vi "write spi file type1.vi"(8 "milliseconds to wait":u32, 11 "addr/data":string[][](array[string])) -> (3 "res":bool)   [LabVIEW 2018]
uses:
  Dll1_x64_191014_0/Dll1_x64_191014_0.lvlib
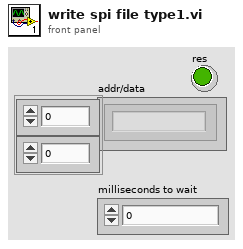
[diagram p1: front panel]
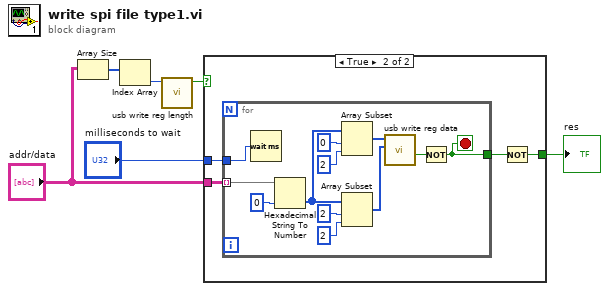
[diagram p0: block diagram]
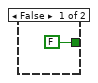
[diagram p2: hidden frame]
diagram:
  n1 = Array Size(array="addr/data") -> (size(s)=w5:i32[])
  n2 = Index Array(array=w5) -> (element=w4:i32)  [unwired: 1 in]
  n3 = call "usb write reg length.vi"("lengthToWrite"=w4) -> ("function return"=w3:bool)  [unwired: 10 in]
  n4 = case shown="True" w3 {
    tunnel: "addr/data" -> [_ w11]
    tunnel: [FALSE w9] -> w2
    tunnel: "milliseconds to wait" -> [_ w8]
    frame False {
    }
    frame True {
      n5 = for {
        tunnel: w11 -> [w17] mode=indexing
        tunnel: [w13] -> w10
        tunnel: w8 -> [w12]
        stop <- w13 stop-if-true
        n6 = Wait (ms)(milliseconds to wait=w12) -> ()  [unwired: 1 out]
        n7 = Hexadecimal String To Number(string=w17, default (0uL)=u32 0 ("default (0 U32)")) -> (number=w18:u32[])  [unwired: 1 in, 1 out]
        n8 = Array Subset(array=w18, index=0, length=2) -> (w15:u32[])
        n9 = Array Subset(array=w18, index=2, length=2) -> (w16:u32[])
        n10 = call "usb write reg data.vi"("write_data"=w16, "addr"=w15) -> ("function return"=w14:bool)  [unwired: 7 in, 2 out]
        n11 = Not(x=w14) -> (.not. x?=w13:bool)
      }
      n12 = Not(x=w10) -> (.not. x?=w9:bool)
    }
  }
  "res" <- w2
